vi "Configure Channel Characteristics.vi"(0 "CS++Scope":refnum<class "CS++Scope.lvclass">, 5 "channel name (\"CHANNEL1\")":string="CHANNEL1", 7 "input impedance (1.0E+6 ohms)":dbl[unit]=1000000.0 format="%.2e", 9 "max input frequency (1.0E+6 Hz)":dbl[unit]=1000000.0 format="%.2e", 11 "error in (no error)":errorcluster) -> (4 "CS++Scope out":refnum<class "CS++Scope.lvclass">, 15 "error out":errorcluster)   [LabVIEW 2013, in "CS++Scope.lvlib" / "CS++Scope.lvclass"]
doc: "This VI configures the properties that control the electrical characteristics of the channel. These properties are the input impedance and the maximum frequency of the input signal."
uses:
  CS++Scope.lvclass
  CSPP_Core/Classes/CS++ProcessVariables/ProcessVariable/PV.lvclass
  PV-Enum-n.ctl
  CS++Scope.lvclass/CS++Scope.ctl
  CSPP_Core/Classes/CS++ProcessVariables/PVConnection/PVConnection.lvclass
  CSPP_Core/Classes/CS++ProcessVariables/ProcessVariable/PV.lvclass/PV.ctl
  CSPP_Core/Classes/CS++ProcessVariables/ProcessVariable/Write Data.vi
  CSPP_Core/Classes/CS++ProcessVariables/ProcessVariable/Write Timestamp.vi
  CSPP_Core/Classes/CS++ProcessVariables/ProcessVariable/Write Quality.vi
  CSPP_Core/Classes/CS++ProcessVariables/ProcessVariable/Write status.vi
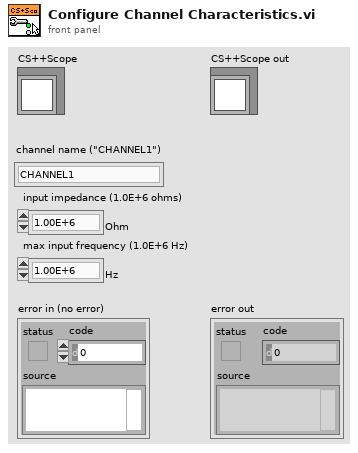
[diagram p1: front panel]
types:
  T1 = typedef "CS++Scope.lvlib/CS++Scope.lvclass/PV-Enum-n.ctl" = enum16{"InputImpedance", "MaxInputFrequency", "VerticalRange", "ProbeAttenuation", "VerticalOffset", "VerticalCoupling", "ChannelEnabled"}
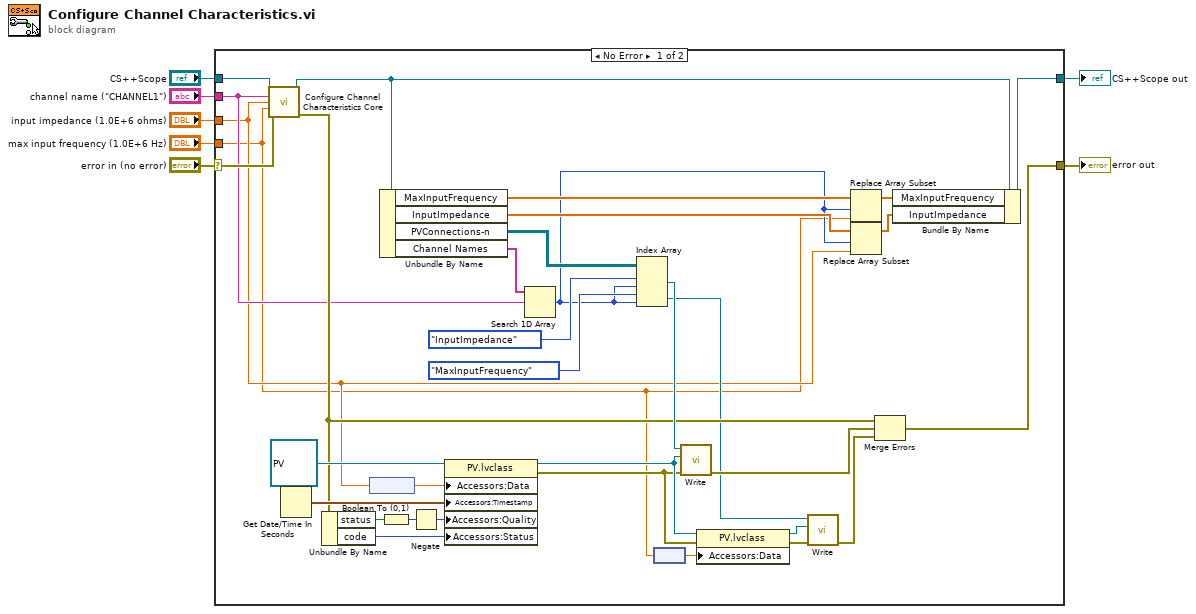
[diagram p0: block diagram]
diagram:
  n1 = case shown="No Error" "error in (no error)" {
    selector: "error in (no error)" -> [w13 w43]
    tunnel: [w14 w43] -> w6
    tunnel: [w15 w42] -> w2
    tunnel: "CS++Scope" -> [w16 w42]
    tunnel: "channel name (\"CHANNEL1\")" -> [w12 _]
    tunnel: "input impedance (1.0E+6 ohms)" -> [w11 _]
    tunnel: "max input frequency (1.0E+6 Hz)" -> [w9 _]
    frame No Error {
      n2 = call-dynamic "Configure Channel Characteristics Core.vi"("CS++Scope"=w16, "channel name (\"CHANNEL1\")"=w12, "input impedance (1.0E+6 ohms)"=w11, "max input frequency (1.0E+6 Hz)"=w9, "error in (no error)"=w13) -> ("CS++Scope out"=w41:refnum<class "CS++Scope.lvclass">, "error out"=w32:errorcluster)  [unwired: 9 in]
      n3 = Get Date/Time In Seconds() -> (seconds since 1Jan1904=w35:timestamp)
      n4 = Unbundle By Name(w32) -> ("status"=w38:bool, "code"=w39:i32)
      n5 = node(w11) -> (w10:dbl)
      n6 = Unbundle By Name(w41) -> ("MaxInputFrequency"=w21:dbl[unit][], "InputImpedance"=w18:dbl[unit][], "PVConnections-n"=w34:refnum<class "PVConnection.lvclass">[][], "Channel Names"=w30:string[])
      n7 = Boolean To (0,1)(Boolean=w38) -> (0, 1=w37:i16)
      n8 = Negate(x=w37) -> (-x=w36:i16)
      n9 = property class="PV.lvclass"(reference=refnum<class "PV.lvclass"> refnum ("CS++ProcessVariables.lvlib:PV.lvclass"), "Accessors:Data"=w10, "Accessors:Timestamp"=w35, "Accessors:Quality"=w36, "Accessors:Status"=w39) -> (reference out=w24:refnum<class "PV.lvclass">, error out=w23:errorcluster)  [unwired: 1 in]
      n10 = Search 1D Array(1D array=w30, element=w12) -> (index of element=w17:i32)  [unwired: 1 in]
      n11 = Index Array(array=w34, index (row) #1=PV-Enum-n."InputImpedance" ("PV-Enum-n"), index (col) #1=w17, index (row) #2=PV-Enum-n."MaxInputFrequency" ("PV-Enum-n"), index (col) #2=w17) -> (element #1=w33:refnum<class "PVConnection.lvclass">, element #2=w25:refnum<class "PVConnection.lvclass">)
      n12 = node(w9) -> (w8:dbl)
      n13 = call-dynamic "Write.vi"("error in (no error)"=w23, "PV"=w24, "PVConnection in"=w33) -> ("error out"=w31:errorcluster)  [unwired: 7 in, 1 out]
      n14 = property class="PV.lvclass"(reference=w24, error in=w23, "Accessors:Data"=w8) -> (reference out=w26:refnum<class "PV.lvclass">, error out=w27:errorcluster)
      n15 = call-dynamic "Write.vi"("error in (no error)"=w27, "PV"=w26, "PVConnection in"=w25) -> ("error out"=w22:errorcluster)  [unwired: 7 in, 1 out]
      n16 = Replace Array Subset(array=w21, new element=w9, index=w17) -> (w20:dbl[unit][])
      n17 = Replace Array Subset(array=w18, new element=w11, index=w17) -> (w19:dbl[unit][])
      n18 = Merge Errors(w32, w31, w22) -> (w14:errorcluster)
      n19 = Bundle By Name(cluster=w41, "MaxInputFrequency"=w20, "InputImpedance"=w19) -> (w15:refnum<class "CS++Scope.lvclass">)
    }
    frame Error {
    }
  }
  "error out" <- w6
  "CS++Scope out" <- w2
